vi "RSZVB Set Mixer Delay LAN Connection.vi"(8 "error in (no error)":errorcluster {"code" format="%.0x"}, 9 "LAN Connection (LAN1)":i32(ring)=1 items=["LAN1"=1, "LAN2"=2], 10 "Channel (1)":i32=1, 11 "VISA session":refnum<visa-resource-name>) -> (0 "error out":errorcluster {"code" format="%.0x"}, 3 "dup VISA session":refnum<visa-resource-name>)   [LabVIEW 2011]
doc: "Selects the LAN connection for the mixer delay measurement with external receiver. The VI has no effect if a single analyzer (internal receiver) is used.\n\nNotes:\n\n(1) This mode requires options R&S ZVA-K9 and R&S ZVA-K4\n\nRemote-control command(s):\n[SENSe<Ch>:]FREQuency:MDELay:RECeiver:USE"
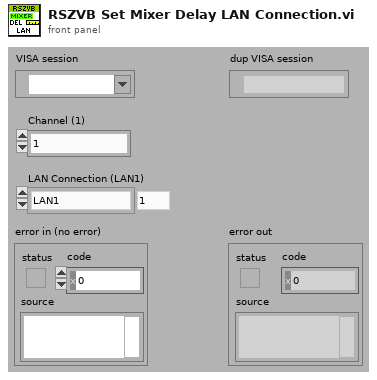
[diagram p1: front panel]
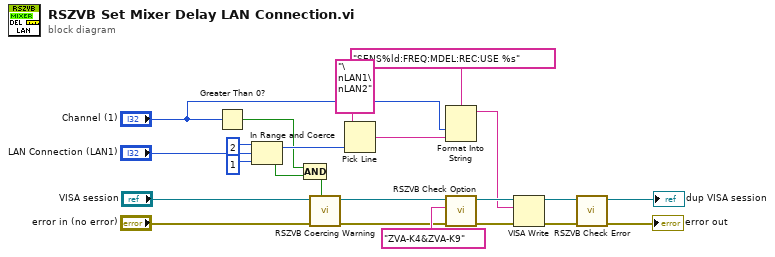
[diagram p0: block diagram]
diagram:
  n1 = Greater Than 0?(x="Channel (1)") -> (x > 0?=w11:bool)
  n2 = In Range and Coerce(upper limit=2, x="LAN Connection (LAN1)", lower limit=1) -> (coerced(x)=w14:i32, In Range?=w12:bool)
  n3 = Compound Arithmetic op=AND(w11, w12) -> (w10:bool)
  n4 = call "RSZVB Coercing Warning.vi"("In Range?"=w10, "error in (no error)"="error in (no error)", "VISA session"="VISA session") -> ("error out"=w7:errorcluster, "dup VISA session"=w8:refnum<visa-resource-name>)  [unwired: 7 in]
  n5 = Pick Line(multi-line string="\nLAN1\nLAN2", line index=w14) -> (output string=w9:string)  [unwired: 1 in]
  n6 = Format Into String(format string="SENS%ld:FREQ:MDEL:REC:USE %s", "Channel (1)", w9) -> (resulting string=w19:string)  [unwired: 2 in, 1 out]
  n7 = call "RSZVB Check Option.vi"("error in (no error)"=w7, "Options"="ZVA-K4&ZVA-K9", "VISA session"=w8) -> ("error out"=w21:errorcluster, "dup VISA session"=w20:refnum<visa-resource-name>)  [unwired: 7 in]
  n8 = VISA Write(VISA resource name=w20, write buffer=w19, error in (no error)=w21) -> (VISA resource name out=w17:refnum<visa-resource-name>, error out=w18:errorcluster)  [unwired: 1 out]
  n9 = call "RSZVB Check Error.vi"("error in (no error)"=w18, "VISA session"=w17) -> ("error out"=→"error out":errorcluster, "dup VISA session"=→"dup VISA session":refnum<visa-resource-name>)  [unwired: 8 in]
